vi "test-1.vi"() -> ()   [LabVIEW 2019]
panel:
  in  "stop":bool
  out "Slide":u8(slide) scale=0.0..100.0
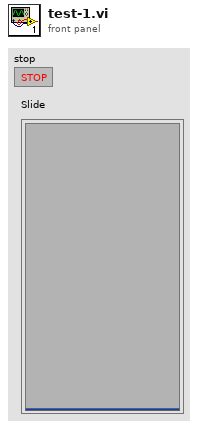
[diagram p1: front panel]
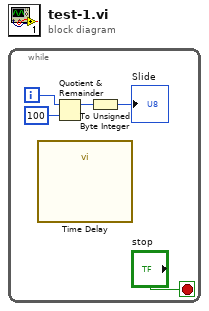
[diagram p0: block diagram]
diagram:
  n1 = while {
    i -> [w5]
    stop <- "stop" stop-if-true
    n2 = call "Time Delay"() -> ()  [unwired: 11 in, 1 out]
    n3 = Quotient & Remainder(x=w5, y=100) -> (x-y*floor(x/y)=w4:i32)  [unwired: 1 out]
    n4 = To Unsigned Byte Integer(number=w4) -> (unsigned 8bit integer=→"Slide":u8)
  }
